vi "OldGetWaypoints.vi"() -> ()   [LabVIEW 2013]
uses:
  <vilib>/Analysis/NI_AALBase.lvlib
  <vilib>/Analysis/baseanly.llb/Unit Vector (DBL).vi
  <vilib>/Analysis/NI_AALPro.lvlib
  <vilib>/Analysis/coordinate.llb/2D Cartesian Coordinate Rotation (Scalar).vi
  Data/TypeDefs/UTM Location.ctl
  Waypoint/Waypoint.lvclass
  RoundBouy/RoundBouy.lvclass
panel:
  in  "Boats Current Position":T1 {"North" format="%#_10f"; "East" format="%#_8f"}
  out "Waypoint Array":refnum<class "Waypoint.lvclass">[](array[class])
  out "RoundBouy out":refnum<class "RoundBouy.lvclass">
  in  "RoundBouy in":refnum<class "RoundBouy.lvclass">
  out "Error Out":errorcluster
  in  "Error In":errorcluster
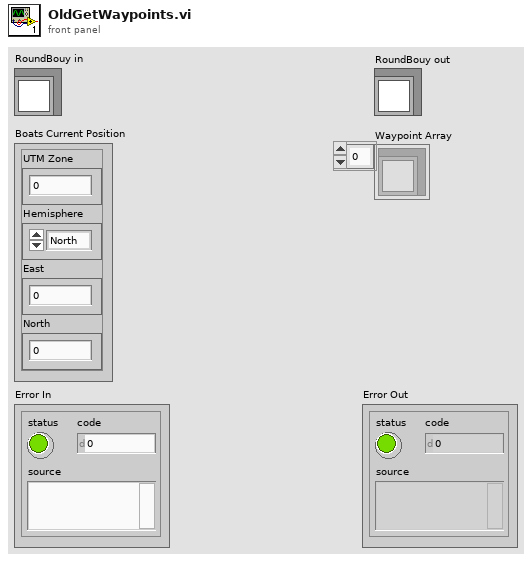
[diagram p1: front panel]
types:
  T1 = typedef "UTM Location.ctl" = cluster{"UTM Zone":dbl, "Hemisphere":enum16{"North", "South"}, "East":dbl, "North":dbl}
  T2 = typedef "MissionTypeControl.ctl" = enum16{"Idle at Point", "Drive to Waypoint", "Round Buoy to Port", "Round Buoy to Starboard", "Pass Between Buoys", "Station Keeping"}
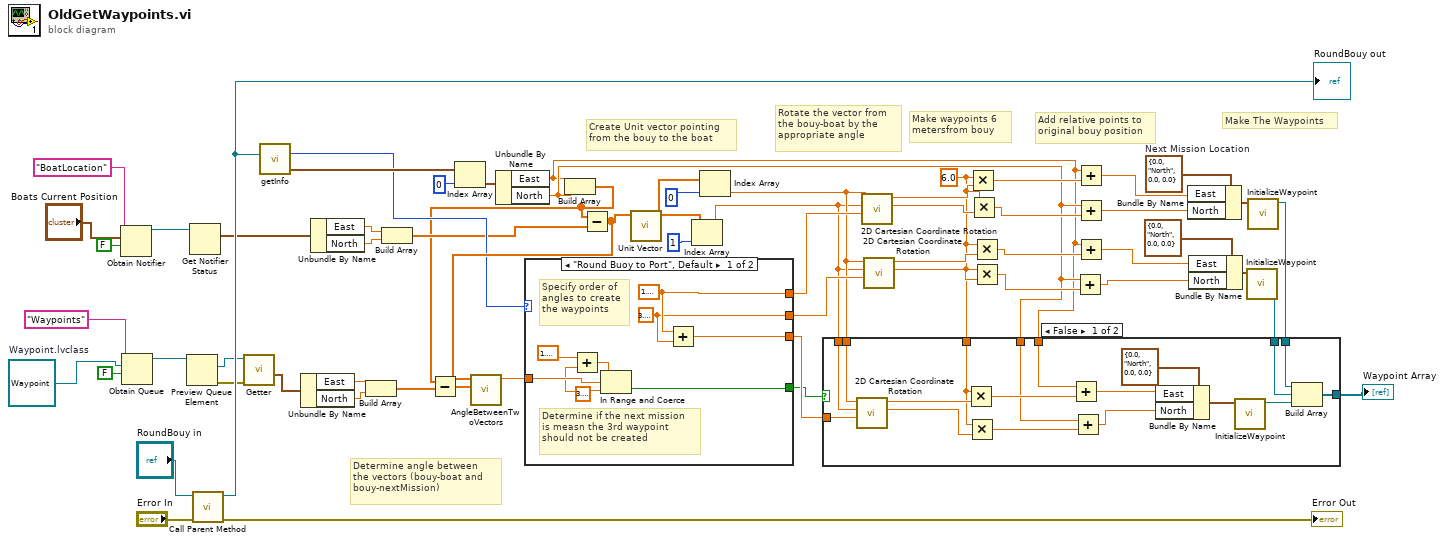
[diagram p0: block diagram]
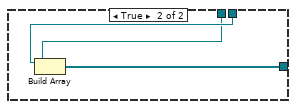
[diagram p2: hidden frame]
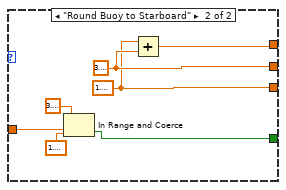
[diagram p3: hidden frame]
diagram:
  w5 = refnum<class "Waypoint.lvclass"> refnum  # Waypoint.lvclass
  w42 = T1 {"UTM Zone"=0.0, "Hemisphere"=enum."North", "East"=0.0, "North"=0.0}  # Next Mission Location
  w21 = 6.0
  # "Create Unit vector pointing \nfrom the bouy to the boat"
  # "Determine angle between \nthe vectors (bouy-boat and \nbouy-nextMission)"
  # "Make The Waypoints"
  # "Rotate the vector from \nthe bouy-boat by the \nappropriate angle"
  # "Make waypoints 6 \nmetersfrom bouy"
  # "Add relative points to \noriginal bouy position"
  n1 = Obtain Notifier(name (unnamed)="BoatLocation", notification data type="Boats Current Position", create if not found? (T)=FALSE) -> (notifier out=w12:refnum<notifier>)  [unwired: 1 in, 2 out]
  n2 = Obtain Queue(name (unnamed)="Waypoints", element data type=w5, create if not found? (T)=FALSE) -> (queue out=w4:refnum<queue>)  [unwired: 2 in, 2 out]
  n3 = Preview Queue Element(queue=w4) -> (element=w2:refnum<class "Waypoint.lvclass">, error out=w3:errorcluster)  [unwired: 2 in, 2 out]
  n4 = Get Notifier Status(notifier=w12) -> (current notification=w8:T1)  [unwired: 1 in, 4 out]
  n5 = call-parent "Call Parent Method"("Error In"="Error In", "GenericMission in"="RoundBouy in") -> ("Error Out"=→"Error Out":errorcluster, "GenericMission out"=w58:refnum<class "RoundBouy.lvclass">)  [unwired: 7 in, 1 out]
  "RoundBouy out" <- w58
  n6 = call "Getter.vi"("Error In"=w3, "Waypoint In"=w2) -> ("Coords"=w1:T1)  [unwired: 4 in, 5 out]
  n7 = call-dynamic "getInfo.vi"("GenericMission in"=w58) -> ("Mission Type"=w25:T2, "Points of Interest"=w26:T1[])  [unwired: 6 in, 7 out]
  n8 = Unbundle By Name(w1) -> ("East"=w47:dbl, "North"=w48:dbl)
  n9 = Unbundle By Name(w8) -> ("East"=w55:dbl, "North"=w54:dbl)
  n10 = Build Array(w47, w48) -> (w46:dbl[])
  n11 = Build Array(w55, w54) -> (w14:dbl[])
  n12 = Index Array(array=w26, index=0) -> (element=w56:T1)
  n13 = Unbundle By Name(w56) -> ("East"=w19:dbl, "North"=w20:dbl)
  n14 = Build Array(w19, w20) -> (w13:dbl[])
  n15 = Subtract(x=w13, y=w46) -> (x-y=w44:dbl[])
  n16 = Subtract(x=w13, y=w14) -> (x-y=w45:dbl[])
  n17 = call "AngleBetweenTwoVectors.vi"("Rotated Vector"=w44, "Base Vector"=w45) -> ("Angle Between Vectors"=w39:dbl)  [unwired: 9 in]
  n18 = case shown="\"Round Buoy to Port\", Default" w25 {
    tunnel: [w69 w75] -> w50
    tunnel: [w68 w76] -> w49
    tunnel: [w67 w74] -> w22
    tunnel: w39 -> [w66 w73]
    tunnel: [w65 w72] -> w15
    frame "Round Buoy to Port", Default {
      w63 = 3.141592653589793
      w68 = 3.141592653589793
      w69 = 1.5707963267948966
      # "Determine if the next mission \nis measn the 3rd waypoint \nshould not be created"
      # "Specify order of \nangles to create \nthe waypoints"
      n19 = Add(x=1.5707963267948966, y=w63) -> (x+y=w64:dbl)
      n20 = In Range and Coerce(upper limit=w64, x=w66, lower limit=w63) -> (In Range?=w65:bool)  [unwired: 1 out]
      n21 = Add(x=w69, y=w68) -> (x+y=w67:dbl)
    }
    frame "Round Buoy to Starboard" {
      w76 = 3.141592653589793
      w74 = 1.5707963267948966
      n22 = In Range and Coerce(upper limit=3.141592653589793, x=w73, lower limit=1.5707963267948966) -> (In Range?=w72:bool)  [unwired: 1 out]
      n23 = Add(x=w74, y=w76) -> (x+y=w75:dbl)
    }
  }
  n24 = call-poly <vilib>:"Unit Vector.vi"("Input Vector"=w45) -> ("Unit Vector"=w53:dbl[])  [unwired: 8 in, 2 out]
  n25 = Index Array(array=w53, index=1) -> (element=w23:dbl)
  n26 = Index Array(array=w53, index=0) -> (element=w24:dbl)
  n27 = call-poly <vilib>:"2D Cartesian Coordinate Rotation.vi"("theta"=w50, "y"=w23, "x"=w24) -> ("y out"=w37:dbl, "x out"=w38:dbl)  [unwired: 6 in, 1 out]
  n28 = call-poly <vilib>:"2D Cartesian Coordinate Rotation.vi"("theta"=w49, "y"=w23, "x"=w24) -> ("y out"=w36:dbl, "x out"=w35:dbl)  [unwired: 6 in, 1 out]
  n29 = Multiply(x=w21, y=w38) -> (x*y=w32:dbl)
  n30 = Multiply(x=w21, y=w37) -> (x*y=w31:dbl)
  n31 = Multiply(x=w21, y=w35) -> (x*y=w30:dbl)
  n32 = Multiply(x=w21, y=w36) -> (x*y=w29:dbl)
  n33 = Add(x=w20, y=w29) -> (x+y=w28:dbl)
  n34 = Add(x=w19, y=w32) -> (x+y=w33:dbl)
  n35 = Add(x=w20, y=w31) -> (x+y=w34:dbl)
  n36 = Add(x=w19, y=w30) -> (x+y=w27:dbl)
  n37 = Bundle By Name(cluster=w42, "East"=w33, "North"=w34) -> (w43:T1)
  n38 = Bundle By Name(cluster=T1 {"UTM Zone"=0.0, "Hemisphere"=enum."North", "East"=0.0, "North"=0.0} ("Next Mission Location"), "East"=w27, "North"=w28) -> (w40:T1)
  n39 = call "InitializeWaypoint.vi"("Coords"=w40) -> ("Waypoint Out"=w18:refnum<class "Waypoint.lvclass">)  [unwired: 10 in]
  n40 = call "InitializeWaypoint.vi"("Coords"=w43) -> ("Waypoint Out"=w17:refnum<class "Waypoint.lvclass">)  [unwired: 10 in]
  n41 = case shown="False" w15 {
    tunnel: [w94 w95] -> w16
    tunnel: w17 -> [w93 w97]
    tunnel: w18 -> [w92 w96]
    tunnel: w22 -> [w88 _]
    tunnel: w24 -> [w87 _]
    tunnel: w23 -> [w86 _]
    tunnel: w21 -> [w83 _]
    tunnel: w19 -> [w78 _]
    tunnel: w20 -> [w77 _]
    frame False {
      n42 = call-poly <vilib>:"2D Cartesian Coordinate Rotation.vi"("theta"=w88, "y"=w86, "x"=w87) -> ("y out"=w85:dbl, "x out"=w84:dbl)  [unwired: 6 in, 1 out]
      n43 = Multiply(x=w83, y=w84) -> (x*y=w79:dbl)
      n44 = Multiply(x=w83, y=w85) -> (x*y=w80:dbl)
      n45 = Add(x=w78, y=w79) -> (x+y=w81:dbl)
      n46 = Add(x=w77, y=w80) -> (x+y=w82:dbl)
      n47 = Bundle By Name(cluster=T1 {"UTM Zone"=0.0, "Hemisphere"=enum."North", "East"=0.0, "North"=0.0} ("Next Mission Location"), "East"=w81, "North"=w82) -> (w91:T1)
      n48 = call "InitializeWaypoint.vi"("Coords"=w91) -> ("Waypoint Out"=w89:refnum<class "Waypoint.lvclass">)  [unwired: 10 in]
      n49 = Build Array(w93, w92, w89) -> (w94:refnum<class "Waypoint.lvclass">[])
    }
    frame True {
      n50 = Build Array(w97, w96) -> (w95:refnum<class "Waypoint.lvclass">[])
    }
  }
  "Waypoint Array" <- w16
